vi "Test shm get Response enter Control LV.vi"(8 "error in (no error)":errorcluster, 11 "ackcmd_Ctl":T1) -> (0 "error out":errorcluster, 2 "function return":i32, 3 "ackcmd_Ctl out":T1)   [LabVIEW 2018, in "SALLV_Test.lvlib"]
doc: "int Test_shm_getResponse_enterControlLV(Test_ackcmdLV *ackcmd_Ctl);"
uses:
  SALLV_Test.lvlib
  SALLV_Test.so
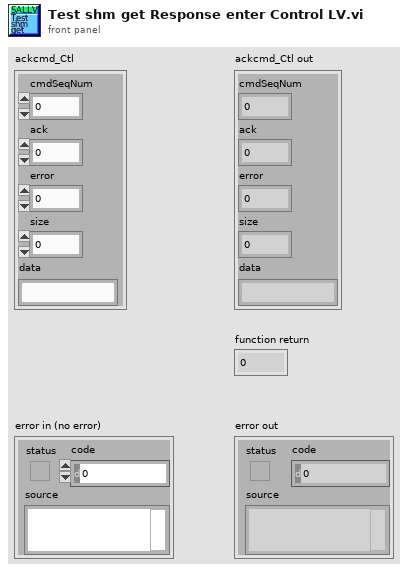
[diagram p1: front panel]
types:
  T1 = cluster{"cmdSeqNum":i32, "ack":i32, "error":i32, "size":i32, "data":string}
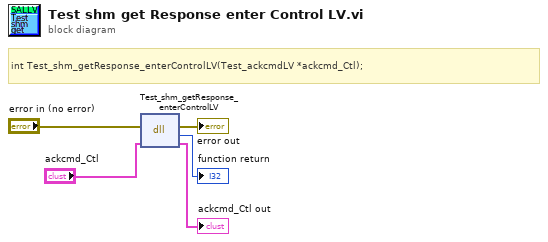
[diagram p0: block diagram]
diagram:
  # "int Test_shm_getResponse_enterControlLV(Test_ackcmdLV *ackcmd_Ctl);"
  n1 = dll-call lib="home/ttsai/Documents/salLabVIEWtestData/SALLV_Test.*" fn="Test_shm_getResponse_enterControlLV"(error in="error in (no error)", "ackcmd_Ctl"="ackcmd_Ctl") -> (error out=→"error out":errorcluster, →"function return":i32, "ackcmd_Ctl"=→"ackcmd_Ctl out":T1)  [unwired: 2 in, 1 out]
